vi "ExecuteCommand.vi"(0 "reference in":refnum<class "DqmhModuleDiagramGraph.lvclass">, 1 "CommandData":variant, 2 "selected":T1, 3 "selectedEdge":refnum<class "AbstractEdge.lvclass">, 4 "SelectedNodes":refnum<class "AbstractNode.lvclass">[](array[class]), 5 "error in (no error)":errorcluster) -> (14 "reference out":refnum<class "DqmhModuleDiagramGraph.lvclass">, 15 "Cancelled":bool, 19 "error out":errorcluster)   [LabVIEW 2016, in "DqmhModuleDiagramGraph.lvclass"]
uses:
  <resource>/Framework/Providers/Open_GDS/UML/DqmhModuleDiagramGraph_class/DqmhModuleDiagramGraph.lvclass
  <resource>/Framework/Providers/Open_GDS/UML/AbstractNode_class/AbstractNode.lvclass
  <resource>/Framework/Providers/Open_GDS/UML/AbstractEdge_class/AbstractEdge.lvclass
  <resource>/Framework/Providers/Open_GDS/UML/UMLEditor/UMLEditor tooltype.ctl
  <resource>/Framework/Providers/Open_GDS/UML/DQMHModuleNode_class/DQMHModuleNode.lvclass
  <resource>/Framework/Providers/Open_GDS/UML/DQMHModuleNode_class/ExternalSetTypes.ctl
  <resource>/Framework/Providers/Open_GDS/UML/DQMH_API_class/DQMH_API.lvclass
panel:
  out "StatusText":string
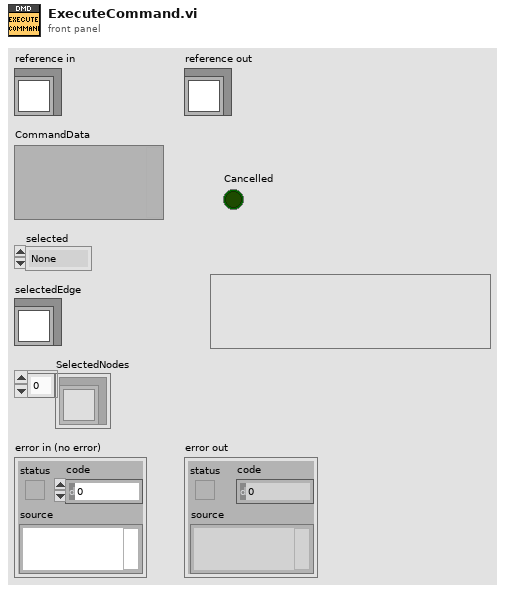
[diagram p1: front panel]
types:
  T1 = typedef "UMLEditor tooltype.ctl" = enum16{"None", "Node", "Edge"}
  T2 = typedef "DQMHModuleNode.lvclass/ExternalSetTypes.ctl" = enum16{"Name", "Attributes", "Methods", "Position", "ShowEvents", "ShowInternalData", "ClassPath"}
  T3 = enum16{"Request", "Broadcast", "Request and Wait for Reply", "Round Trip"}
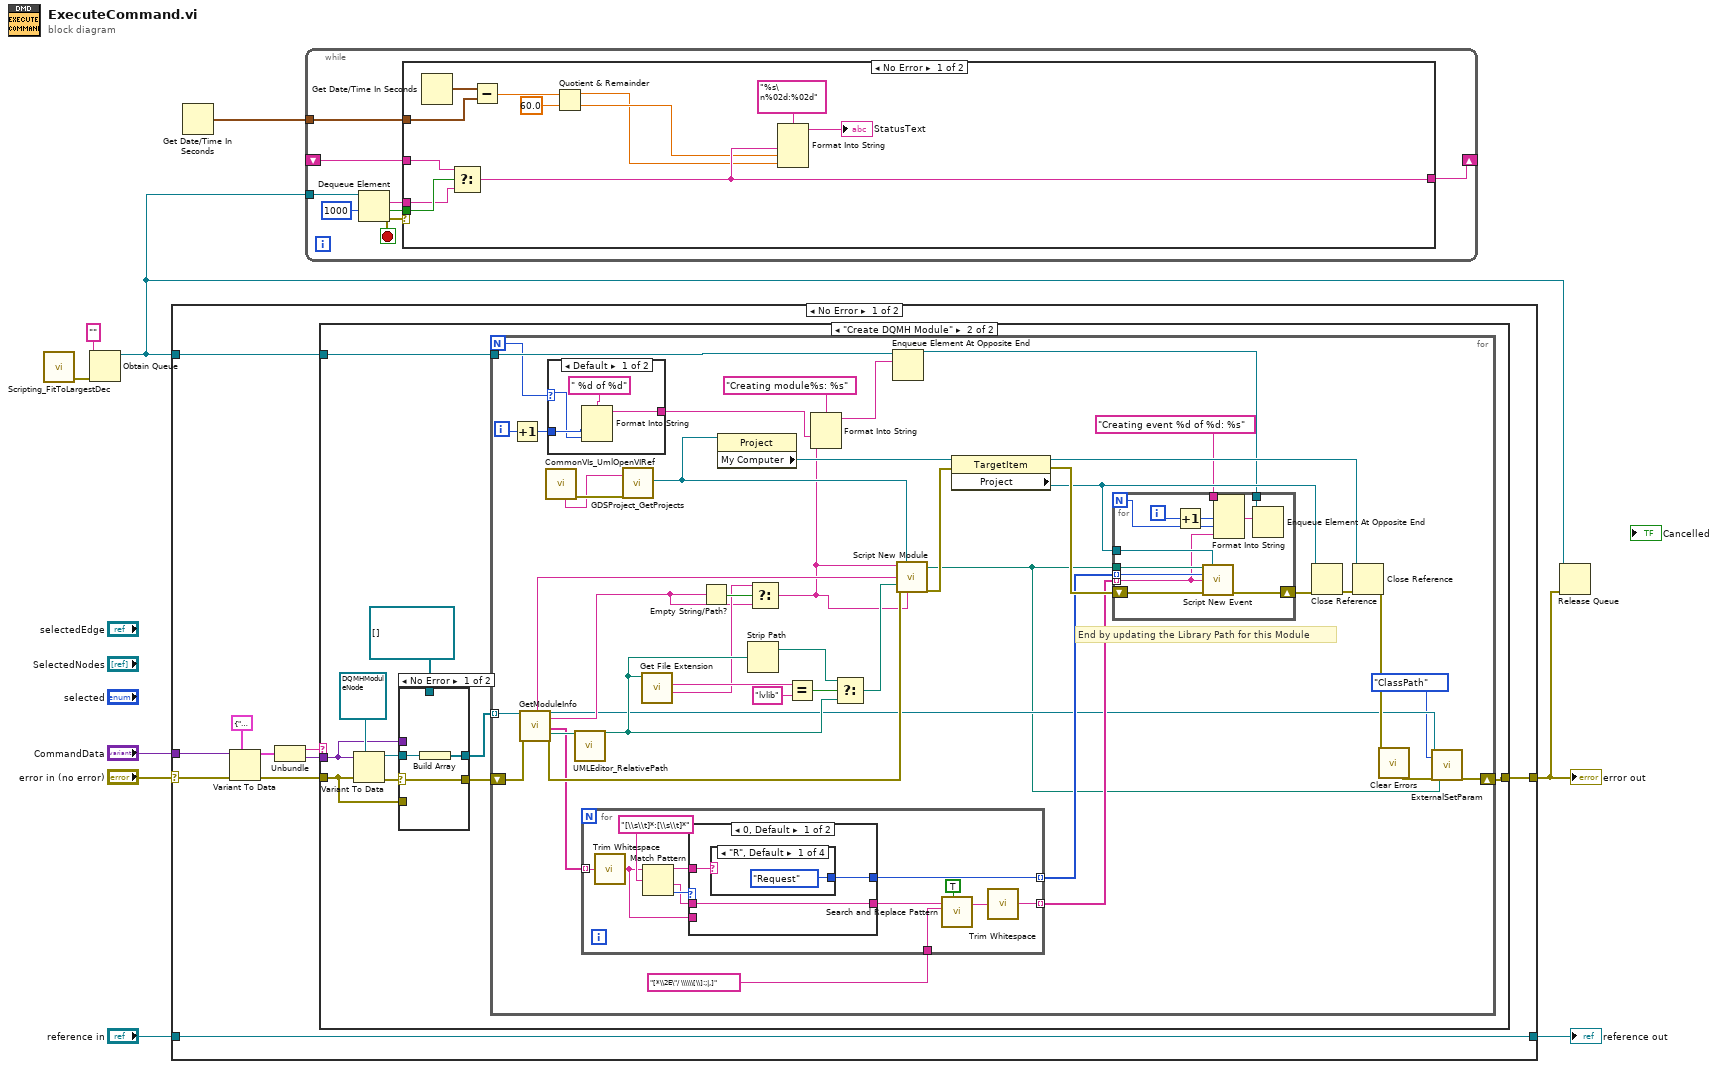
[diagram p0: block diagram]
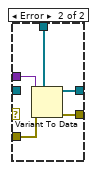
[diagram p4: hidden frame]
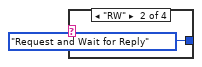
[diagram p6: hidden frame]
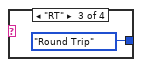
[diagram p7: hidden frame]
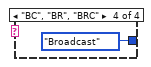
[diagram p8: hidden frame]
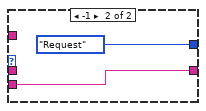
[diagram p9: hidden frame]
diagram:
  n1 = call <resource>:"Scripting_FitToLargestDec.vi"() -> ("error out"=w5:errorcluster)  [unwired: 6 in, 1 out]
  n2 = Obtain Queue(element data type="" ("y"), error in (no error)=w5) -> (queue out=w3:refnum<queue>)  [unwired: 3 in, 2 out]
  n3 = case shown="No Error" "error in (no error)" {
    selector: "error in (no error)" -> [w16 w121]
    tunnel: [w12 w121] -> w4
    tunnel: [w19 w120] -> w7
    tunnel: "reference in" -> [w19 w120]
    tunnel: "CommandData" -> [w17 _]
    tunnel: w3 -> [w10 _]
    frame No Error {
      n4 = Variant To Data(error in=w16, type=cluster{"Cmd":string, "Data":variant} {"Cmd"="", "Data"=variant} ("FlattenCommandSettings"), Variant=w17) -> (data=w15:cluster{"Cmd":string, "Data":variant}, error out=w13:errorcluster)
      n5 = Unbundle(w15) -> ("Cmd"=w14:string, "Data"=w11:variant)
      n6 = case shown="\"Create DQMH Module\"" w14 {
        tunnel: w13 -> [w20 w21]
        tunnel: [w20 w28] -> w12
        tunnel: w11 -> [_ w22]
        tunnel: w10 -> [_ w27]
        frame Default {
        }
        frame "Create DQMH Module" {
          n7 = Variant To Data(error in=w21, type=refnum<class "DQMHModuleNode.lvclass"> refnum ("DQMHModuleNode"), Variant=w22) -> (data=w29:refnum<class "DQMHModuleNode.lvclass">, error out=w25:errorcluster)
          n8 = case shown="No Error" w25 {
            selector: w25 -> [w31 _]
            tunnel: w29 -> [w33 _]
            tunnel: [w32 w34] -> w26
            tunnel: [w31 w35] -> w24
            tunnel: refnum<class "DQMHModuleNode.lvclass">[] [] -> [_ w38]
            tunnel: w22 -> [_ w37]
            tunnel: w21 -> [_ w36]
            frame No Error {
              n9 = Build Array(w33) -> (w32:refnum<class "DQMHModuleNode.lvclass">[])
            }
            frame Error {
              n10 = Variant To Data(error in=w36, type=w38, Variant=w37) -> (data=w34:refnum<class "DQMHModuleNode.lvclass">[], error out=w35:errorcluster)
            }
          }
          n11 = for {
            N -> [w48]
            tunnel: w27 -> [w50]
            tunnel: w26 -> [w49] mode=indexing
            shift-right: [w42] -> w28
            shift-left: w24 -> [w81]
            i -> [w46]
            # "End by updating the Library Path for this Module"
            n12 = Increment(x=w46) -> (x+1=w47:i32)
            n13 = call-dynamic "GetModuleInfo.vi"("reference in"=w49, "error in (no error)"=w81) -> ("Template"=w78:string, "reference out"=w41:refnum<class "DQMHModuleNode.lvclass">, "ModuleName"=w70:string, "Events"=w59:string[], "ModulePath"=w82:path, "error out"=w71:errorcluster)  [unwired: 6 in, 6 out]
            n14 = call <resource>:"CommonVIs_UmlOpenVIRef.vi"() -> ("error out"=w69:errorcluster, "ProjectNameOut"=w68:string)  [unwired: 4 in, 6 out]
            n15 = case shown="Default" w48 {
              selector: w48 -> [w84 _]
              tunnel: w47 -> [w85 _]
              tunnel: [w83 _] -> w45
              frame Default {
                n16 = Format Into String(format string=" %d of %d" ("element"), w85, w84) -> (resulting string=w83:string)  [unwired: 2 in, 1 out]
              }
              frame 1 {
              }
            }
            n17 = call <resource>:"UMLEditor_RelativePath.vi"("Path In"=w82) -> ("ConvertToAbsolutePath(If possible)"=w76:path)  [unwired: 1 in, 17 out]
            n18 = for {
              tunnel: w59 -> [w98] mode=indexing
              tunnel: [w87] -> w58 mode=indexing
              tunnel: [w95] -> w57 mode=indexing
              tunnel: "[*\\2E\"/ \\\\\\[\\]:;|,]" ("regular expression") -> [w88]
              n19 = call <vilib>:"Trim Whitespace.vi"("string"=w98) -> ("trimmed string"=w92:string)  [unwired: 1 in]
              n20 = Match Pattern(string=w92, regular expression="[\\s\\t]*:[\\s\\t]*") -> (before substring=w94:string, after substring=w93:string, offset past match=w96:i32)  [unwired: 1 in, 1 out]
              n21 = case shown="0, Default" w96 {
                tunnel: w93 -> [w99 _]
                tunnel: [w99 w106] -> w91
                tunnel: [w100 T3."Request" ("Event Type")] -> w95
                tunnel: w94 -> [w101 _]
                tunnel: w92 -> [_ w106]
                frame 0, Default {
                  n22 = case shown="\"R\", Default" w101 {
                    tunnel: [T3."Request" ("Event Type") T3."Request and Wait for Reply" ("Event Type") T3."Round Trip" ("Event Type") T3."Broadcast" ("Event Type")] -> w100
                    frame "R", Default {
                    }
                    frame "RW" {
                    }
                    frame "RT" {
                    }
                    frame "BC", "BR", "BRC" {
                    }
                  }
                }
                frame -1 {
                }
              }
              n23 = call <vilib>:"Search and Replace Pattern.vi"("string"=w91, "regular expression (\"\")"=w88, "replace all? (F)"=TRUE) -> ("result string"=w90:string)  [unwired: 2 in, 1 out]
              n24 = call <vilib>:"Trim Whitespace.vi"("string"=w90) -> ("trimmed string"=w87:string)  [unwired: 1 in]
            }
            n25 = call <resource>:"GDSProject_GetProjects.vi"("GetProjectRefByName"=w68, "error in (no error)"=w69) -> ("Project Refnum"=w67:refnum<vi>)  [unwired: 1 in, 16 out]
            n26 = call <vilib>:"Get File Extension.vi"("file"=w76) -> ("filename without extension"=w72:string, "lowercase file extension"=w80:string)  [unwired: 6 in, 3 out]
            n27 = Empty String/Path?(string/path=w70) -> (empty?=w73:bool)
            n28 = property class="Project"(reference=w67) -> ("My Computer"=w66:refnum<vi>)  [unwired: 1 in, 2 out]
            n29 = Strip Path(path=w76) -> (stripped path=w75:path)  [unwired: 1 out]
            n30 = Select(t=w72, s=w73, f=w70) -> (s? t:f=w54:string)
            n31 = Equal?(x=w80, y="lvlib") -> (x = y?=w77:bool)
            n32 = Format Into String(format string="Creating module%s: %s" ("element"), w45, w54) -> (resulting string=w55:string)  [unwired: 2 in, 1 out]
            n33 = Select(t=w75, s=w77, f=w76) -> (s? t:f=w74:path)
            n34 = Enqueue Element At Opposite End(queue=w50, element=w55) -> (queue out=w51:refnum<queue>)  [unwired: 2 in, 2 out]
            n35 = call <resource>:"Script New Module.vi"("Module Name"=w54, "Project"=w67, "ModuleType(String)"=w78, "Module Save Path"=w74, "error in (no error)"=w71, "Line 1 text"=w54) -> ("ModulePath(lvlib)"=w39:path, "error out"=w64:errorcluster)  [unwired: 8 in]
            n36 = property class="TargetItem"(reference=w66, error in=w64) -> (reference out=w63:refnum<vi>, error out=w65:errorcluster, "Project"=w60:refnum<vi>)
            n37 = for {
              N -> [w110]
              tunnel: w60 -> [w117]
              tunnel: w39 -> [w116]
              shift-right: [w118] -> w62
              shift-left: w65 -> [w119]
              tunnel: w58 -> [w113] mode=indexing
              tunnel: w57 -> [w115] mode=indexing
              tunnel: "Creating event %d of %d: %s" ("element") -> [w114]
              tunnel: w51 -> [w111]
              i -> [w109]
              n38 = Increment(x=w109) -> (x+1=w108:i32)
              n39 = call <resource>:"Script New Event.vi"("LibraryPath"=w116, "Project"=w117, "Event Type"=w115, "Event Name"=w113, "error in (no error)"=w119) -> ("error out"=w118:errorcluster)  [unwired: 9 in, 1 out]
              n40 = Format Into String(format string=w114, w108, w110, w113) -> (resulting string=w112:string)  [unwired: 2 in, 1 out]
              n41 = Enqueue Element At Opposite End(queue=w111, element=w112) -> ()  [unwired: 2 in, 3 out]
            }
            n42 = Close Reference(reference=w60, error in (no error)=w62) -> (error out=w61:errorcluster)
            n43 = Close Reference(reference=w63, error in (no error)=w61) -> (error out=w52:errorcluster)
            n44 = call <vilib>:"Clear Errors.vi"("error in (no error)"=w52) -> ("error out"=w43:errorcluster)  [unwired: 5 in, 1 out]
            n45 = call-dynamic "ExternalSetParam.vi"("reference in"=w41, "setParameter"=ExternalSetTypes."ClassPath", "error in (no error)"=w43, "ClassPath"=w39) -> ("error out"=w42:errorcluster)  [unwired: 14 in, 1 out]
          }
        }
      }
    }
    frame Error {
    }
  }
  "error out" <- w4
  "reference out" <- w7
  n46 = Get Date/Time In Seconds() -> (seconds since 1Jan1904=w1:timestamp)
  n47 = while {
    tunnel: w3 -> [w129]
    tunnel: w1 -> [w126]
    shift-right: [w122] -> _
    shift-left: _ -> [w123]
    stop <- w128 stop-if-true
    n48 = Dequeue Element(queue=w129, timeout in ms (-1)=1000) -> (element=w125:string, timed out?=w124:bool, error out=w128:errorcluster)  [unwired: 1 in, 1 out]
    n49 = case shown="No Error" w128 {
      tunnel: w126 -> [w140 _]
      tunnel: w125 -> [w137 _]
      tunnel: w124 -> [w139 _]
      tunnel: w123 -> [w138 _]
      tunnel: [w135 _] -> w122
      frame No Error {
        n50 = Get Date/Time In Seconds() -> (seconds since 1Jan1904=w141:timestamp)
        n51 = Select(t=w138, s=w139, f=w137) -> (s? t:f=w135:string)
        n52 = Subtract(x=w141, y=w140) -> (x-y=w134:dbl)
        n53 = Quotient & Remainder(x=w134, y=60.0) -> (x-y*floor(x/y)=w131:dbl, floor(x/y)=w132:dbl)
        n54 = Format Into String(format string="%s\n%02d:%02d", w135, w132, w131) -> (resulting string=→"StatusText":string)  [unwired: 2 in, 1 out]
      }
      frame Error {
      }
    }
  }
  n55 = Release Queue(queue=w3, error in (no error)=w4) -> ()  [unwired: 1 in, 3 out]
